vi "update.vi"(0 "reference in":refnum<class "ForecastConditionDisplay.lvclass">, 2 "WeatherData":T1, 5 "error in (no error)":errorcluster) -> (14 "reference out":refnum<class "ForecastConditionDisplay.lvclass">, 19 "error out":errorcluster)   [LabVIEW 2020, in "ForecastConditionDisplay.lvclass"]
uses:
  ForecastConditionDisplay.lvclass
  WeatherData.ctl
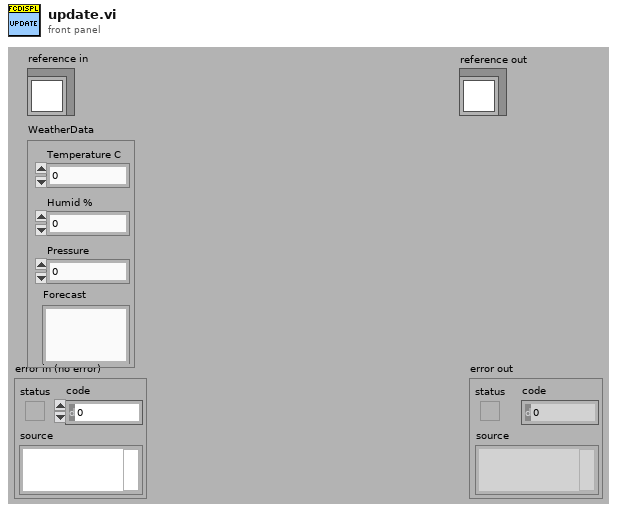
[diagram p1: front panel]
types:
  T1 = typedef "WeatherData.ctl" = cluster{"Temperature C":dbl, "Humid %":dbl, "Pressure":dbl, "Forecast":string}
  T2 = typedef "ForecastConditionDisplay.lvclass/ObjectAttributes.ctl" = cluster{"WeatherData":T1}
  T3 = typedef "CurrentConditionDisplay.lvclass/ObjectAttributes.ctl" = cluster{"WeatherData":T1}
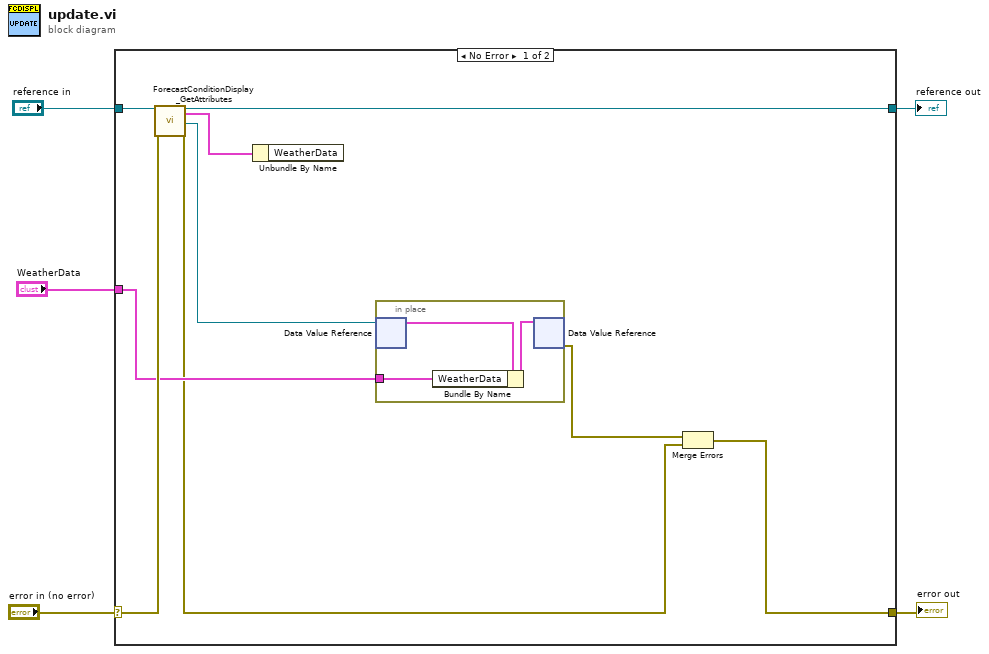
[diagram p0: block diagram]
diagram:
  n1 = case shown="No Error" "error in (no error)" {
    selector: "error in (no error)" -> [w14 w19]
    tunnel: [w6 w19] -> w4
    tunnel: [w11 w18] -> w2
    tunnel: "reference in" -> [w12 w18]
    tunnel: "WeatherData" -> [w8 _]
    frame No Error {
      n2 = call "ForecastConditionDisplay_GetAttributes.vi"("reference in"=w12, "error in (no error)"=w14) -> ("reference out"=w11:refnum<class "ForecastConditionDisplay.lvclass">, "Data"=w13:T2, "DataRef"=w9:refnum<data-value>, "error out"=w7:errorcluster)  [unwired: 14 in]
      n3 = Unbundle By Name(w13) -> ()  [unwired: 1 out]
      n4 = in-place {
        in-place-border: w8 -> [w15]
        n5 = in-place-dvr #1(w9) -> (w17:T3)  [unwired: 1 out]
        n6 = Bundle By Name(cluster=w17, "WeatherData"=w15) -> (w16:T3)
        n7 = in-place-dvr #1(w16) -> (w10:errorcluster)  [unwired: 1 out]
      }
      n8 = Merge Errors(w10, w7) -> (w6:errorcluster)
    }
    frame Error {
    }
  }
  "error out" <- w4
  "reference out" <- w2
